vi "Trap2.vi"(0 "Heizen?Trap2":bool, 2 "Per[us]Trap2":u32 caption="PerTrap2[us]", 5 "PIDTrap2":T1 {"proportional gain (Kc)" format="%.11g"; "integral gain (Kc*Ts/Ti)" format="%.11g"; "derivative gain (Kc*Td/Ts)" format="%.11g"}, 7 "UTempMaxTrap2":fxp<+/-,16,4> format="%.14g", 9 "UWidrMaxTrap2":fxp<+/-,16,4> format="%.14g", 11 "UTempSPTrap2":fxp<+/-,16,4> format="%.14g", 13 "warten[us]Trap2":u32=200) -> (4 "UTemp[V]Trap2":fxp<+/-,16,4> format="%.25g", 15 "UWidr[V]Trap2":fxp<+/-,16,4> format="%.25g")   [LabVIEW 2010]
uses:
  <vilib>/eio/EIONode/EIONode.xnode
  <vilib>/rvi/eio/nirviEIOImplementation/nirviEIOImplementation.xnode
  <vilib>/rvi/eio/common/nirviEmuClasses.ctl
  <vilib>/addons/control/pid/fpga.llb/XNode/niFpgaPID.xnode
  <vilib>/rvi/eio/common/nirviEmuTemplateMethod_noerrors.vi
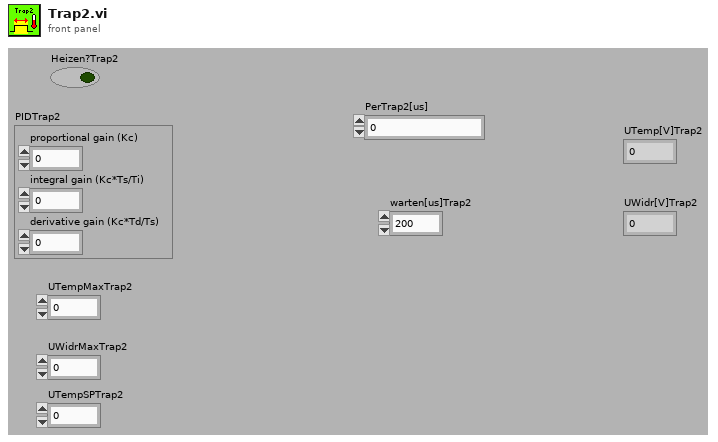
[diagram p1: front panel]
types:
  T1 = cluster{"proportional gain (Kc)":fxp<+/-,16,8>, "integral gain (Kc*Ts/Ti)":fxp<+/-,16,8>, "derivative gain (Kc*Td/Ts)":fxp<+/-,16,8>}
  T2 = cluster{"output high":fxp<+/-,16,4>, "output low":fxp<+/-,16,4>}
  T3 = typedef "nirviEmuClasses.ctl" = enum16{"IO Read", "IO Write", "Method", "Property Read", "Property Write"}
  T4 = cluster{"proportional gain (Kc)":i16, "integral gain (Kc*Ts/Ti)":i16, "derivative gain (Kc*Td/Ts)":i16}
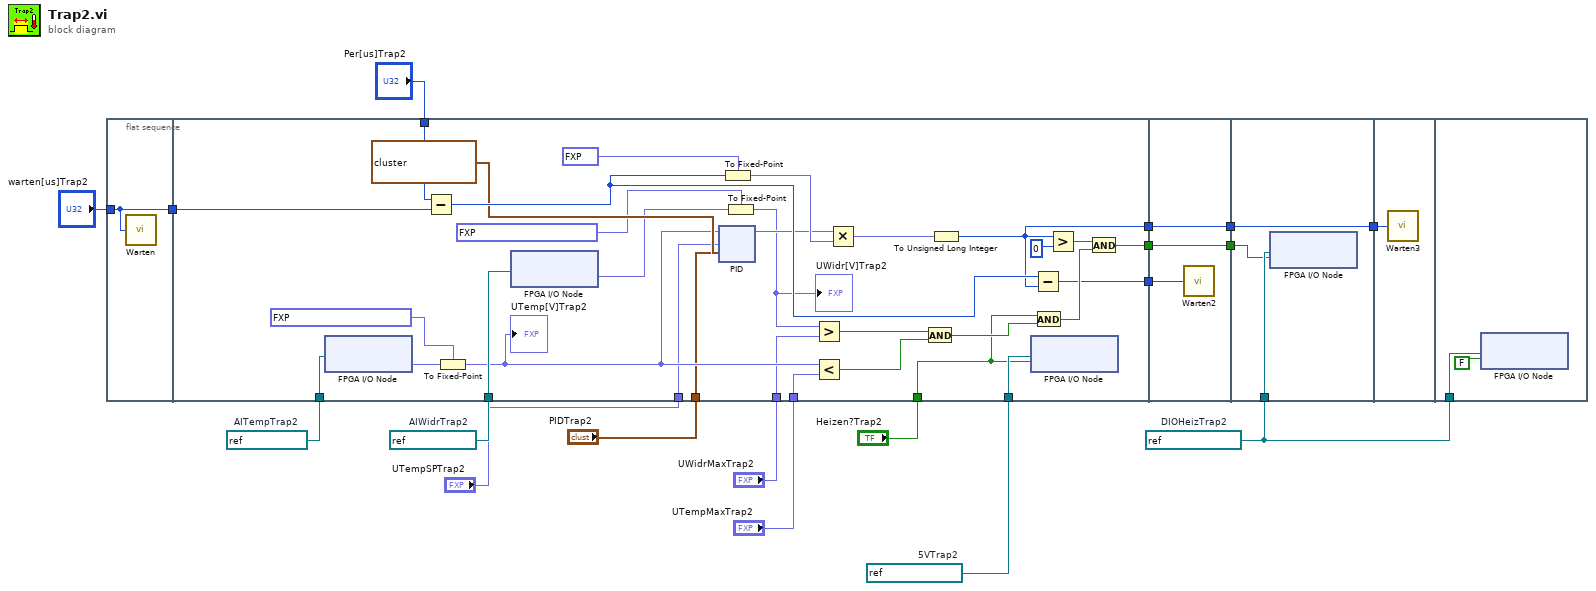
[diagram p0: block diagram]
diagram:
  w9 = refnum<k21> "Mod1/AI31"  # AIWidrTrap2
  w8 = refnum<k21> "Mod1/AI1"  # AITempTrap2
  w7 = refnum<k21> "Mod6/DIO18"  # DIOHeizTrap2
  w6 = refnum<k21> "Mod6/DIO20"  # 5VTrap2
  n1 = flat-sequence {
    tunnel: [w19] -> w18
    tunnel: "warten[us]Trap2" -> [w19]
    tunnel: w8 -> [w50]
    tunnel: w9 -> [w49]
    tunnel: [w42] -> w17
    tunnel: w18 -> [w33]
    tunnel: [w40] -> w16
    tunnel: [w39] -> w15
    tunnel: "Per[us]Trap2" -> [w26]
    tunnel: w6 -> [w25]
    tunnel: "PIDTrap2" -> [w24]
    tunnel: "UTempMaxTrap2" -> [w23]
    tunnel: "UWidrMaxTrap2" -> [w22]
    tunnel: "Heizen?Trap2" -> [w21]
    tunnel: "UTempSPTrap2" -> [w20]
    tunnel: [w138] -> w14
    tunnel: w17 -> [w138]
    tunnel: [w137] -> w13
    tunnel: w16 -> [w137]
    tunnel: w15 -> [w136]
    tunnel: w7 -> [w141]
    tunnel: w14 -> [w140]
    tunnel: [w139] -> w12
    tunnel: w13 -> [w139]
    tunnel: w12 -> [w153]
    tunnel: w7 -> [w155]
    frame #0 {
      n2 = call "Warten"("Count(uSec)"=w19) -> ()  [unwired: 1 out]
    }
    frame #1 {
      n3 = xnode "FPGA I/O Node"("FPGA I/O In"=w50) -> ("I/O Item"=w28:fxp<+/-,26,5>)  [unwired: 1 out]
      n4 = Subtract(x=w26, y=w33) -> (x-y=w41:u32)
      n5 = To Fixed-Point(fixed-point type=fxp<+/-,16,4> 0.0 ("Festkommatyp"), number=w28) -> (fixed-point=w27:fxp<+/-,16,4>)
      "UTemp[V]Trap2" <- w27
      n6 = xnode "FPGA I/O Node"("FPGA I/O In"=w49) -> ("I/O Item"=w31:fxp<+/-,26,5>)  [unwired: 1 out]
      n7 = xnode ("PID")("process variable"=w27, "setpoint"=w20, "PID gains"=w24, "output range"=T2 {"output high"=1.0, "output low"=0.0}) -> ("output"=w34:fxp<+/-,16,4>)  [unwired: 1 in]
      n8 = To Fixed-Point(fixed-point type=fxp<+/-,21,21> 32768.0 ("output high"), number=w41) -> (fixed-point=w37:fxp<+/-,21,21>)
      n9 = To Fixed-Point(fixed-point type=fxp<+/-,16,4> 0.0 ("Festkommatyp"), number=w31) -> (fixed-point=w30:fxp<+/-,16,4>)
      "UWidr[V]Trap2" <- w30
      n10 = Greater?(x=w30, y=w22) -> (0:w38:bool)
      n11 = Less?(x=w27, y=w23) -> (x < y?=w48:bool)
      n12 = Multiply(x=w34, y=w37) -> (x*y=w36:fxp<+/-,37,25>)
      n13 = And(x=w38, y=w48) -> (x .and. y?=w47:bool)
      n14 = To Unsigned Long Integer(number=w36) -> (unsigned 32bit integer=w40:u32)
      n15 = xnode "FPGA I/O Node"("I/O Item"=w21, "FPGA I/O In"=w25) -> ()  [unwired: 1 out]
      n16 = Subtract(x=w41, y=w40) -> (x-y=w39:u32)
      n17 = And(x=w21, y=w47) -> (x .and. y?=w43:bool)
      n18 = Greater?(x=w40, y=u32 0) -> (0:w44:bool)
      n19 = And(x=w44, y=w43) -> (x .and. y?=w42:bool)
    }
    frame #2 {
      n20 = call "Warten2"("Count(uSec)"=w136) -> ()  [unwired: 1 out]
    }
    frame #3 {
      n21 = xnode "FPGA I/O Node"("I/O Item"=w140, "FPGA I/O In"=w141) -> ()  [unwired: 1 out]
    }
    frame #4 {
      n22 = call "Warten3"("Count(uSec)"=w153) -> ()  [unwired: 1 out]
    }
    frame #5 {
      n23 = xnode "FPGA I/O Node"("I/O Item"=FALSE, "FPGA I/O In"=w155) -> ()  [unwired: 1 out]
    }
  }
